vi "Save Data (SubVI).vi"(4 "Channel":u8, 5 "timestamp":u32, 6 "error in (no error)":errorcluster, 9 "App Data":T1={"Core"={"Current VI Reference"=refnum, "Close Panel on Exit?"=FALSE}, "Delay Positions"=[], "Position Index"=-1, "Shutter Open"=TRUE, "Save File Reference"=refnum, "In Backstep"=FALSE, "Backstep"=FALSE}) -> (0 "error out":errorcluster, 3 "App Data Out":T1={"Core"={"Current VI Reference"=refnum, "Close Panel on Exit?"=FALSE}, "Delay Positions"=[], "Position Index"=-1, "Shutter Open"=TRUE, "Save File Reference"=refnum, "In Backstep"=FALSE, "Backstep"=FALSE})   [LabVIEW 2020]
uses:
  App Data.ctl
  SP200-DQMH/Libraries/SP200/SP200.lvlib
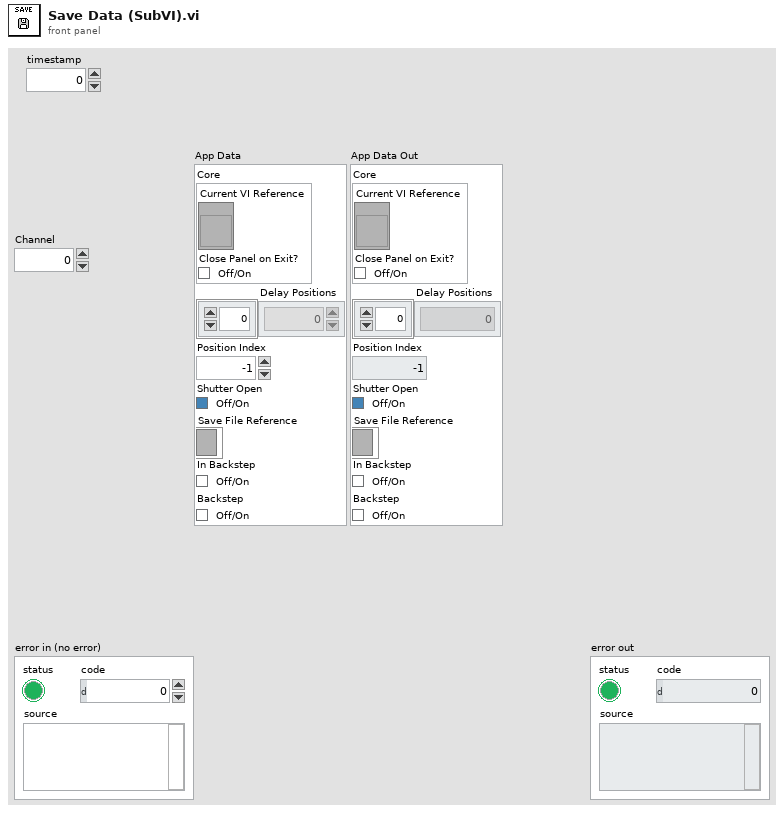
[diagram p1: front panel]
types:
  T1 = typedef "App Data.ctl" = cluster{"Core":cluster{"Current VI Reference":refnum<vi>, "Close Panel on Exit?":bool}, "Delay Positions":dbl[], "Position Index":i32, "Shutter Open":bool, "Save File Reference":refnum<file>, "In Backstep":bool, "Backstep":bool}
  T2 = typedef "SP200.lvlib/Get Data (Reply Payload)--cluster.ctl" = cluster{"Continue Acquiring":bool, "Get Data_error":errorcluster, "Data":dbl[][], "Current values":cluster{"State":i32, "MemFilled":i32, "TimeBase":sgl, " Ewe":sgl, " EweRangeMin":sgl, " EweRangeMax":sgl, "Ece":sgl, "EceRangeMin":sgl, "EceRangeMax":sgl, "Eoverflow":i32, "I":sgl, "IRange":i32, "Ioverflow":i32, "ElapsedTime":sgl, "Freq":sgl, "Rcomp":sgl, "Saturation":sgl, "OptErr":i32, "OptPos":i32}}
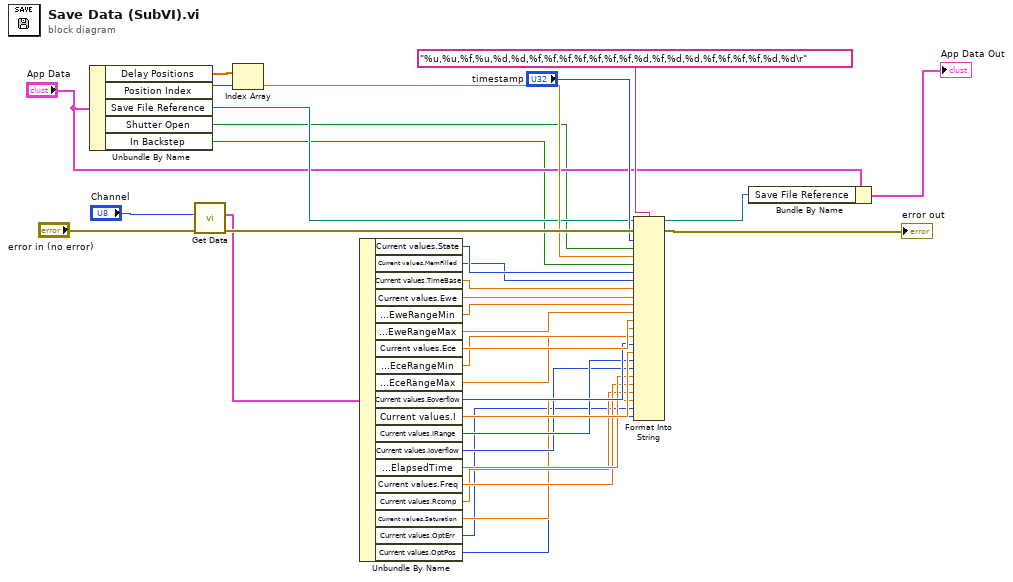
[diagram p0: block diagram]
diagram:
  n1 = Unbundle By Name("App Data") -> ("Delay Positions"=w29:dbl[], "Position Index"=w28:i32, "Save File Reference"=w26:refnum<file>, "Shutter Open"=w2:bool, "In Backstep"=w1:bool)
  n2 = call "Get Data.vi"("error in (no error)"="error in (no error)", "Channel"="Channel") -> ("error out"=w34:errorcluster, "Reply Payload"=w33:T2)  [unwired: 7 in, 1 out]
  n3 = Index Array(array=w29, index=w28) -> (element=w27:dbl)
  n4 = Unbundle By Name(w33) -> ("Current values.State"=w25:i32, "Current values.MemFilled"=w24:i32, "Current values.TimeBase"=w23:sgl, "Current values.Ewe"=w22:sgl, "Current values.EweRangeMin"=w21:sgl, "Current values.EweRangeMax"=w20:sgl, "Current values.Ece"=w19:sgl, "Current values.EceRangeMin"=w18:sgl, "Current values.EceRangeMax"=w17:sgl, "Current values.Eoverflow"=w16:i32, "Current values.I"=w15:sgl, "Current values.IRange"=w14:i32, "Current values.Ioverflow"=w13:i32, "Current values.ElapsedTime"=w12:sgl, "Current values.Freq"=w11:sgl, "Current values.Rcomp"=w10:sgl, "Current values.Saturation"=w9:sgl, "Current values.OptErr"=w8:i32, "Current values.OptPos"=w7:i32)
  n5 = Format Into String(format string="%u,%u,%f,%u,%d,%d,%f,%f,%f,%f,%f,%f,%f,%d,%f,%d,%d,%f,%f,%f,%f,%d,%d\r", initial string=w26, error in=w34, "timestamp", w2, w27, w1, w25, w24, w23, w22, w21, w20, w19, w18, w17, w16, w15, w14, w13, w12, w11, w10, w9, w8, w7) -> (resulting string=w6:refnum<file>, error out=→"error out":errorcluster)
  n6 = Bundle By Name(cluster="App Data", "Save File Reference"=w6) -> (→"App Data Out":T1)
